vi "Read Acquisition State.vi"(0 "device session in":refnum<class "Device Session.lvclass">, 11 "error in":errorcluster) -> (4 "device session out":refnum<class "Device Session.lvclass">, 6 "acquisition state":T1, 8 "data overflow":bool, 10 "samples written":u64, 14 "time elapsed (s)":dbl, 15 "error out":errorcluster)   [LabVIEW 2015, in "Device Session.lvclass"]
doc: "Reads the state of the acquisition engine on the FPGA.\n\n<B>Input Parameters</B>\n\n<B>device session in</B> is a reference to the session containing sessions to all instrument design libraries used in this sample project. This parameter is obtained from the 'Open Session' VI.\n\n<B>error in</B> describes error conditions that occur before this node runs. This input provides standard 'error in' functionality.\n\n<B>Output Parameters</B>\n\n<B>device session out</B> passes a reference to the session to the next VI.\n\n<B>acquisition state</B> returns the current state of the acquisition state machine.\n\n<B>data overflow</B> indicates that a data sample has exceeded the number of allowed bits.\n\n<B>samples written</B> returns the number of samples per channel acquired during the current acquisition.\n\n<B>time elapsed (s)</B> returns the amount of time elapsed during the current acquisition.\n\n<B>error out</B> contains error information. This output provides standard 'error out' functionality."
uses:
  Device Session.lvclass
  Acquisition State.ctl
  Device Session.lvclass/Device Session.ctl
  FPGA Refnum.ctl
  <vilib>/Utility/error.llb/Error Cluster From Error Code.vi
  <vilib>/rvi/errors/niLvFpgaAdjustHostInterfaceError.vi
  <vilib>/rvi/interface/nirviReadWriteControl/nirviReadWriteControl.xnode
  NiFpgaLv.dll
  <vilib>/rvi/interface/Simulation/niFpgaSimulationCallBeginRW.vi
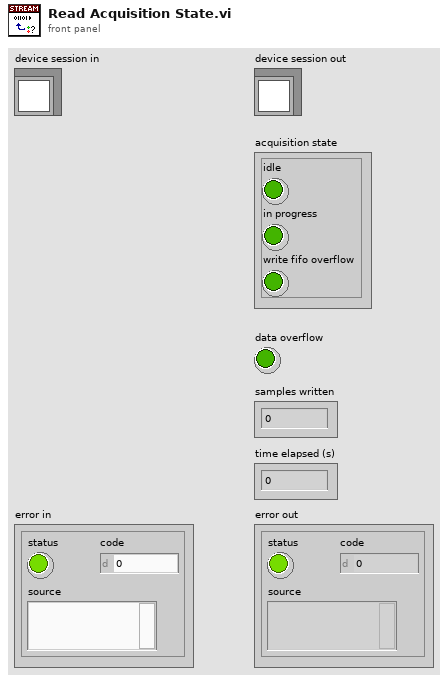
[diagram p1: front panel]
types:
  T1 = typedef "Device Session.lvclass/Acquisition State.ctl" = cluster{"idle":bool, "in progress":bool, "write fifo overflow":bool}
  T2 = cluster{"idle":bool, "in progress":bool, "write fifo overflow":bool}
  T3 = typedef "Device Session.lvclass/FPGA Refnum.ctl" = refnum<k20>
  T4 = typedef "Device Session.lvclass/Device Session Object.ctl" = cluster{"ni5171R FPGA Reference":T3, "niHSAI config":refnum<class "niHSAI Config v1 Host.lvclass">, "configured scaling coefficients":cluster{"gain":dbl, "offset":dbl}[], "number of channels to stream":u8, "selected acq channels":bool[], "number of channels":u32, "actual channel configuration":T5[], "configured channels":bool[], "sample clock rate (Hz)":dbl}
  T5 = typedef "niHSAI Types v1 Host.lvlib/Channel Configuration.ctl" = cluster{"channel":u32, "coupling":T6, "impedance":T7, "bandwidth":T8, "vertical range":dbl, "vertical offset":dbl}
  T6 = typedef "niHSAI Types v1 Host.lvlib/Coupling.ctl" = enum8{"Default", "DC", "AC"}
  T7 = typedef "niHSAI Types v1 Host.lvlib/Impedance.ctl" = enum8{"Default", "1 mega ohm", "50 ohm"}
  T8 = typedef "niHSAI Types v1 Host.lvlib/Bandwidth.ctl" = enum8{"Default", "Full Bandwidth", "Anti-alias Filter"}
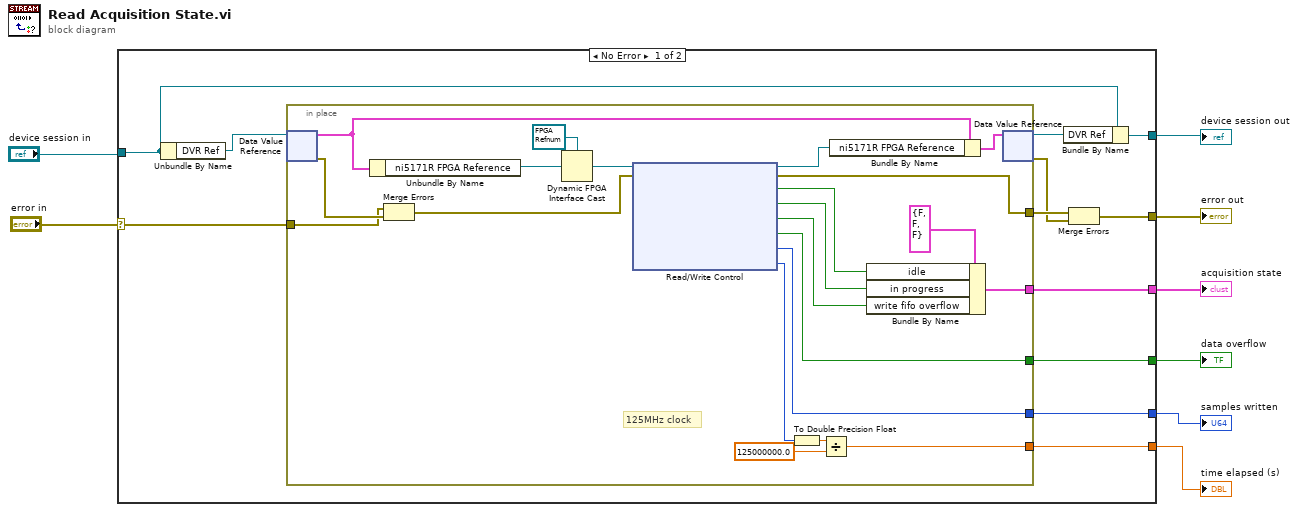
[diagram p0: block diagram]
diagram:
  n1 = case shown="No Error" "error in" {
    selector: "error in" -> [w20 w43]
    tunnel: [w15 w43] -> w5
    tunnel: "device session in" -> [w17 w42]
    tunnel: [w16 w42] -> w6
    tunnel: [w12 _] -> w4
    tunnel: [w11 _] -> w3
    tunnel: [w10 _] -> w2
    tunnel: [w9 _] -> w1
    frame No Error {
      n2 = Unbundle By Name(w17) -> ("DVR Ref"=w19:refnum<data-value>)
      n3 = in-place {
        in-place-border: w20 -> [w39]
        in-place-border: [w36] -> w14
        in-place-border: [w27] -> w12
        in-place-border: [w26] -> w11
        in-place-border: [w25] -> w10
        in-place-border: [w21] -> w9
        # "125MHz clock"
        n4 = in-place-dvr #1(w19) -> (w41:T4, w40:errorcluster)
        n5 = Unbundle By Name(w41) -> ("ni5171R FPGA Reference"=w33:T3)
        n6 = Merge Errors(w39, w40) -> (w38:errorcluster)
        n7 = Dynamic FPGA Interface Cast(Session In=T3 refnum ("FPGA Interface"), Type=w33) -> (Session Out=w32:T3)
        n8 = xnode "Read/Write Control"("FPGA VI Reference In"=w32, "error in"=w38) -> ("FPGA VI Reference Out"=w37:T3, "error out"=w36:errorcluster, "acq.idle"=w29:bool, "acq.in progress"=w30:bool, "acq.fifo overflow"=w31:bool, "data overflow"=w26:bool, "status.samples acquired"=w25:u64, "status.clock cycles"=w23:u64)
        n9 = To Double Precision Float(number=w23) -> (double precision float=w24:dbl)
        n10 = Divide(x=w24, y=125000000.0) -> (x/y=w21:dbl)
        n11 = Bundle By Name(cluster=w41, "ni5171R FPGA Reference"=w37) -> (w35:T4)
        n12 = Bundle By Name(cluster=T2 {"idle"=FALSE, "in progress"=FALSE, "write fifo overflow"=FALSE} ("acquisition state"), "idle"=w29, "in progress"=w30, "write fifo overflow"=w31) -> (w27:T2)
        n13 = in-place-dvr #1(w35) -> (w18:refnum<data-value>, w13:errorcluster)
      }
      n14 = Bundle By Name(cluster=w17, "DVR Ref"=w18) -> (w16:refnum<class "Device Session.lvclass">)
      n15 = Merge Errors(w14, w13) -> (w15:errorcluster)
    }
    frame Error {
    }
  }
  "device session out" <- w6
  "error out" <- w5
  "acquisition state" <- w4
  "data overflow" <- w3
  "samples written" <- w2
  "time elapsed (s)" <- w1
